vi "file header.vi"(8 "error in (no error)":errorcluster, 11 "Error log in":refnum<class "Error log.lvclass">) -> (0 "error out":errorcluster, 3 "Error log out":refnum<class "Error log.lvclass">)   [LabVIEW 2018, in "Error log.lvclass"]
uses:
  Error log.lvclass
  C:/Users/Denis/Desktop/S4CCS/S4CCS/Log File/CCS_Log File.lvclass
  Log File/CCS_Log File.lvclass/CCS_Log File.ctl
  Log File/CCS_Log File.lvclass
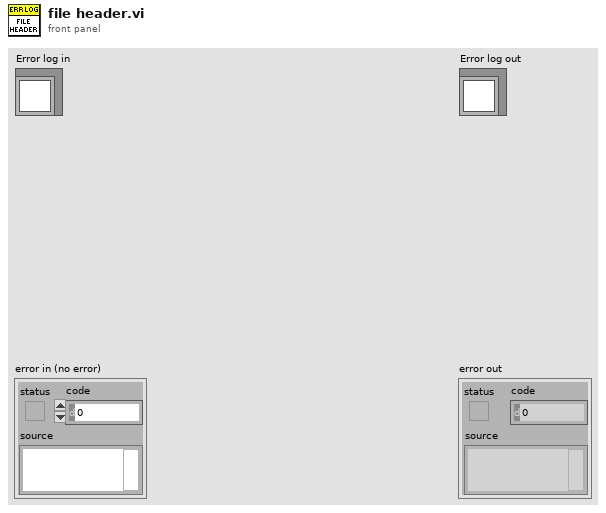
[diagram p1: front panel]
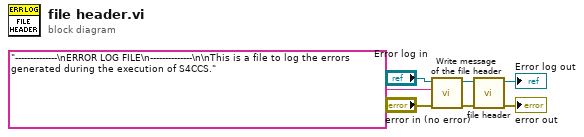
[diagram p0: block diagram]
diagram:
  n1 = call "Write message of the file header.vi"("error in (no error)"="error in (no error)", "message of the file header"="--------------\nERROR LOG FILE\n--------------\n\nThis is a file to log the errors generated during the execution of S4CCS.", "Log File in"="Error log in") -> ("error out"=w4:errorcluster, "Log File out"=w5:refnum<class "Error log.lvclass">)  [unwired: 7 in]
  n2 = call-parent "file header.vi"("error in (no error)"=w4, "Log File in"=w5) -> ("error out"=→"error out":errorcluster, "Log File out"=→"Error log out":refnum<class "Error log.lvclass">)  [unwired: 8 in]
